vi "Execute.Initialize.vi"(8 "error in (no error)":errorcluster, 11 "Cluster":T1={"Events.State"=refnum, "Events.Test Result"=refnum, "Events.Progress"=refnum, "INI.Settings"={"Build Location"=path "C:/Simple Sequence Editor/SequenceRepo", "LoggingLocation"=path "", "Sequence.AbortChannel"="", "Sequence.IterationInfoChannel"="", "Sequence.DurationChannel"="", "Sequence.StepInfoChannel"="", "Sequence.SkipChannel"="", "PlotChannels"=[], "Sequence.InitializeScript"=path "C:/Simple Sequence Editor/SequenceRepo", "Sequence.CleanupScript"=path "", "Log.DefaultRate"=0.0}, "NIVS.AlarmManager"=refnum, "NIVS.BaseLogPath"=path "", "NIVS.DataLogManagerRef"=refnum, "NIVS.DataLogSpecRef"=refnum, "NIVS.Deployed"=FALSE, "NIVS.Events"={"SequenceEvent"=refnum, "SystemChangeEvent"=refnum, "WorkspaceEvent"=refnum}, "NIVS.GatewayIPAddress"="", "NIVS.DataLogGUID"="", "NIVS.ProfileCallback"=refnum, "NIVS.ProfileRef"=refnum, "NIVS.SequenceState"=enum."Idle", "NIVS.SystemDefinitionFile"=path "", "NIVS.SystemStateRefs"={"CustDatRef"=refnum, "EvtRef"=refnum, "Target State User Event"=refnum}, "NIVS.WorkspaceManager"=refnum, "NIVS.EventLogGUID"="", "NIVS.EventLogManagerRef"=refnum, "NIVS.EventLogSpecRef"=refnum, "NIVS.BaseToolPath"=path "", "Restart.Path"=path "", "Sequence.#ofColumns"=0, "Sequence.Iterations"=0, "Sequence.Channels"=[], "Sequence.ValidConfig?"=FALSE, "Station.ID"="", "UDP.Queue"=refnum, "UI.Abort"=refnum, "UI.Alarms"=refnum, "UI.Apply"=refnum, "UI.Back"=refnum, "UI.BaseFileName"=refnum, "UI.CurrentIteration"=refnum, "UI.CurrentStep"=refnum, "UI.CyclicFrequency"=refnum, "UI.Description"=refnum, "UI.DelayTime"=refnum, "UI.DisableAlarms"=refnum, "UI.Duration"=refnum, "UI.EnableLogging"=refnum, "UI.EnableState"=refnum, "UI.High"=refnum, "UI.LogChannels"=refnum, "UI.Low"=refnum, "UI.MonitoredVariable"=refnum, "UI.Next"=refnum, "UI.NumberOfCycles"=refnum, "UI.OperatorName"=refnum, "UI.Pause"=refnum, "UI.Profile"=refnum, "UI.Revert"=refnum, "UI.Skip"=refnum, "UI.Start"=refnum, "UI.StartIteration"=refnum, "UI.StartStep"=refnum, "UI.TabControl"=refnum, "UI.TotalIterations"=refnum, "UI.WaveformDefinition"=refnum, "UI.WaveformPreview"=refnum, "UI.WorkOrderNumber"=refnum, "UI.Chart"=refnum, "UI.Status"=refnum, "UI.DataView"=refnum, "UI.Table"=refnum, "UI.Multihead"=refnum, "UI.ToolTab"=refnum, "UI.Result"=refnum, "UI.Log Path"=refnum, "UI.ReportPath"=refnum, "UI.RestartPath"=refnum, "UI.AlarmLog"=refnum}) -> (0 "error out":errorcluster)   [LabVIEW 2015, in "Single Station Execution.lvlib"]
uses:
  Single Station Execution.lvlib
  Types/Main.StateVariables.ctl
  Types/INI.Settings.ctl
  <vilib>/NI Veristand/Execution/AlarmManager/AlarmManagerAPI.ctl
  NationalInstruments.VeriStand.ClientAPI
  <vilib>/NI Veristand/Execution/DataLogging/IDataLogging Ref.ctl
  <vilib>/NI Veristand/Execution/DataLogging/DataLoggingSpecification Ref.ctl
  Types/Execute.UserEventRefs.ctl
  <vilib>/NI Veristand/Execution/Workspace/SystemStateRegEventRef.ctl
  <vilib>/NI Veristand/Execution/Workspace/Target State Info.ctl
  <vilib>/NI Veristand/Execution/Workspace/Target State.ctl
  Types/Execution.SequenceState.ctl
  <vilib>/NI Veristand/Execution/Workspace/SystemStateEventRef.ctl
  <vilib>/NI Veristand/Execution/Workspace/WorkspaceAPI.ctl
  Types/UDPEngine.QueueCluster.ctl
  Types/UDPEngine.State.ctl
  <vilib>/NI Veristand/Execution/Workspace/NI_VS Workspace ExecutionAPI.lvlib
  <vilib>/NI Veristand/Execution/DataLogging/NI_VS Data Logging API.lvlib
  NationalInstruments.VeriStand.RealTimeSequenceDefinitionApi
  <vilib>/NI Veristand/Execution/AlarmManager/NI_VS AlarmManager ExecutionAPI.lvlib
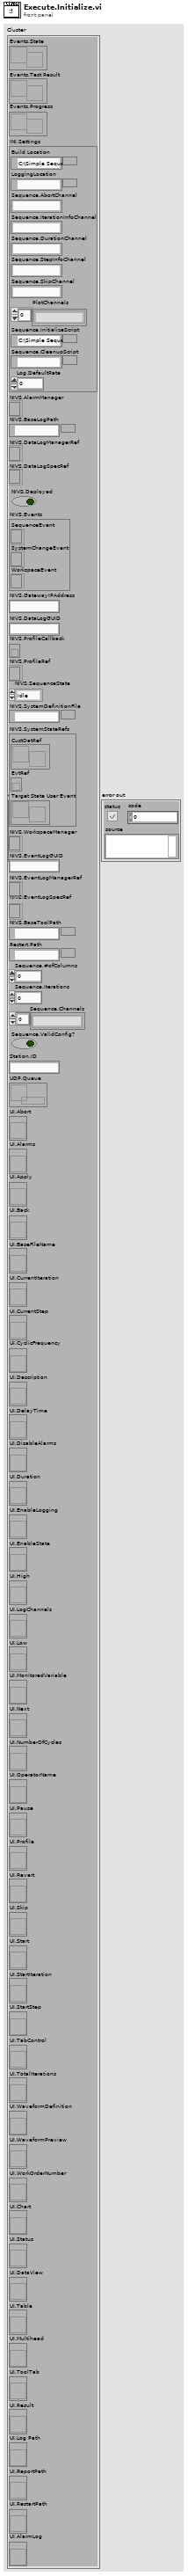
[diagram p1: front panel]
types:
  T1 = typedef "Single Station Execution.lvlib/Main.StateVariables.ctl" = cluster{"Events.State":refnum<user-event>, "Events.Test Result":refnum<user-event>, "Events.Progress":refnum<user-event>, "INI.Settings":T2, "NIVS.AlarmManager":T3, "NIVS.BaseLogPath":path, "NIVS.DataLogManagerRef":T4, "NIVS.DataLogSpecRef":T5, "NIVS.Deployed":bool, "NIVS.Events":T6, "NIVS.GatewayIPAddress":string, "NIVS.DataLogGUID":string, "NIVS.ProfileCallback":refnum<k27>, "NIVS.ProfileRef":refnum<k24>, "NIVS.SequenceState":T8, "NIVS.SystemDefinitionFile":path, "NIVS.SystemStateRefs":T9, "NIVS.WorkspaceManager":T10, "NIVS.EventLogGUID":string, "NIVS.EventLogManagerRef":T4, "NIVS.EventLogSpecRef":T5, "NIVS.BaseToolPath":path, "Restart.Path":path, "Sequence.#ofColumns":i32, "Sequence.Iterations":u32, "Sequence.Channels":string[], "Sequence.ValidConfig?":bool, "Station.ID":string, "UDP.Queue":refnum<queue>, "UI.Abort":refnum<vi>, "UI.Alarms":refnum<vi>, "UI.Apply":refnum<vi>, "UI.Back":refnum<vi>, "UI.BaseFileName":refnum<vi>, "UI.CurrentIteration":refnum<vi>, "UI.CurrentStep":refnum<vi>, "UI.CyclicFrequency":refnum<vi>, "UI.Description":refnum<vi>, "UI.DelayTime":refnum<vi>, "UI.DisableAlarms":refnum<vi>, "UI.Duration":refnum<vi>, "UI.EnableLogging":refnum<vi>, "UI.EnableState":refnum<vi>, "UI.High":refnum<vi>, "UI.LogChannels":refnum<vi>, "UI.Low":refnum<vi>, "UI.MonitoredVariable":refnum<vi>, "UI.Next":refnum<vi>, "UI.NumberOfCycles":refnum<vi>, "UI.OperatorName":refnum<vi>, "UI.Pause":refnum<vi>, "UI.Profile":refnum<vi>, "UI.Revert":refnum<vi>, "UI.Skip":refnum<vi>, "UI.Start":refnum<vi>, "UI.StartIteration":refnum<vi>, "UI.StartStep":refnum<vi>, "UI.TabControl":refnum<vi>, "UI.TotalIterations":refnum<vi>, "UI.WaveformDefinition":refnum<vi>, "UI.WaveformPreview":refnum<vi>, "UI.WorkOrderNumber":refnum<vi>, "UI.Chart":refnum<vi>, "UI.Status":refnum<vi>, "UI.DataView":refnum<vi>, "UI.Table":refnum<vi>, "UI.Multihead":refnum<vi>, "UI.ToolTab":refnum<vi>, "UI.Result":refnum<vi>, "UI.Log Path":refnum<vi>, "UI.ReportPath":refnum<vi>, "UI.RestartPath":refnum<vi>, "UI.AlarmLog":refnum<vi>}
  T2 = typedef "Single Station Execution.lvlib/INI.Settings.ctl" = cluster{"Build Location":path, "LoggingLocation":path, "Sequence.AbortChannel":string, "Sequence.IterationInfoChannel":string, "Sequence.DurationChannel":string, "Sequence.StepInfoChannel":string, "Sequence.SkipChannel":string, "PlotChannels":string[], "Sequence.InitializeScript":path, "Sequence.CleanupScript":path, "Log.DefaultRate":dbl}
  T3 = typedef "NI_VS AlarmManager ExecutionAPI.lvlib/AlarmManagerAPI.ctl" = refnum<k24>
  T4 = typedef "NI_VS Data Logging API.lvlib/IDataLogging Ref.ctl" = refnum<k24>
  T5 = typedef "NI_VS Data Logging API.lvlib/DataLoggingSpecification Ref.ctl" = refnum<k24>
  T6 = typedef "Single Station Execution.lvlib/Execute.UserEventRefs.ctl" = cluster{"SequenceEvent":refnum<event-registration>, "SystemChangeEvent":T7, "WorkspaceEvent":refnum<event-registration>}
  T7 = typedef "NI_VS Workspace ExecutionAPI.lvlib/SystemStateRegEventRef.ctl" = refnum<event-registration>
  T8 = typedef "Single Station Execution.lvlib/Execution.SequenceState.ctl" = enum16{"Idle", "Initializing", "Running", "Paused", "Finalizing", "Complete"}
  T9 = typedef "NI_VS Workspace ExecutionAPI.lvlib/SystemStateEventRef.ctl" = cluster{"CustDatRef":refnum<user-event>, "EvtRef":refnum<k27>, "Target State User Event":refnum<user-event>}
  T10 = typedef "NI_VS Workspace ExecutionAPI.lvlib/WorkspaceAPI.ctl" = refnum<k24>
  T11 = enum8{"Enabled", "Disabled", "Disabled and Grayed Out"}
  T12 = enum16{"Channels (No System Channel)", "Aliases", "All"}
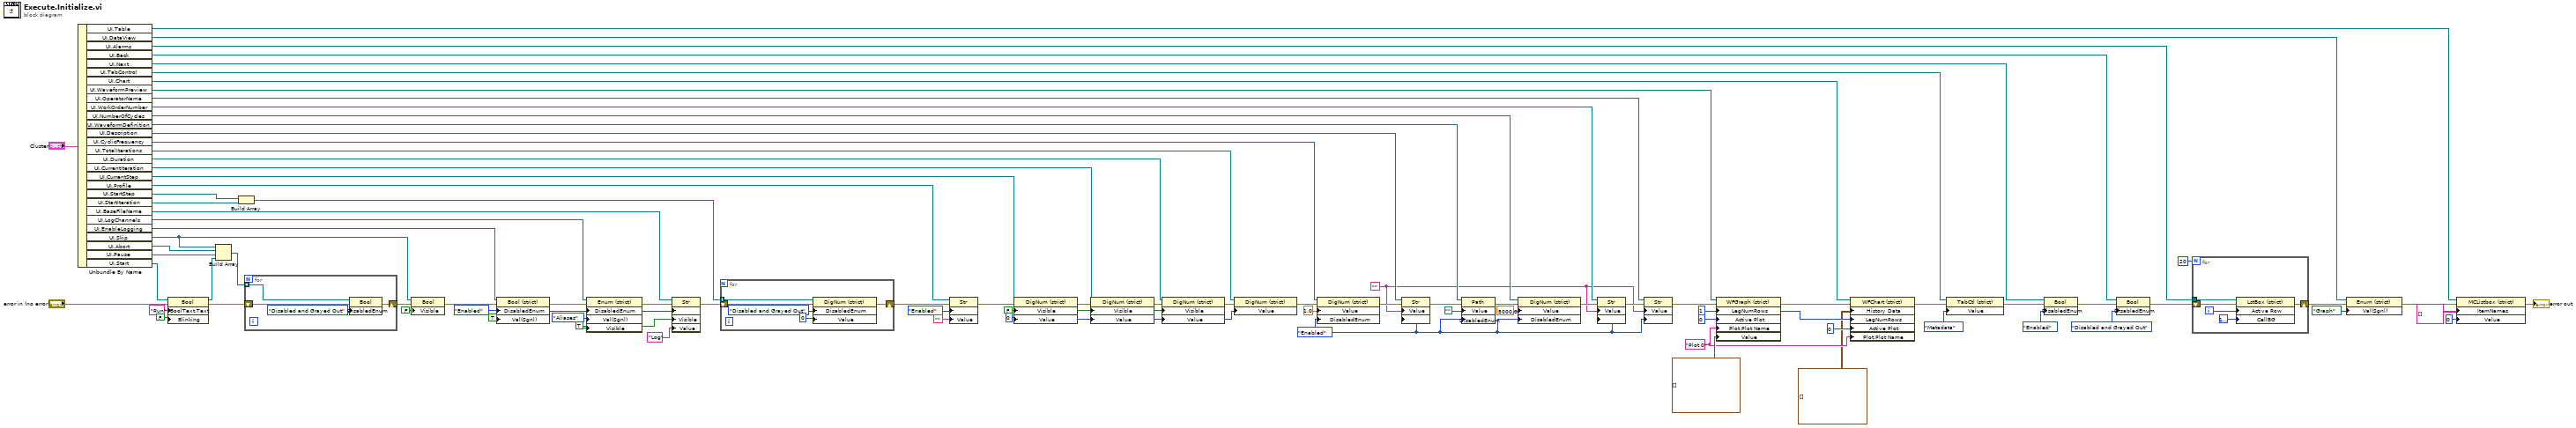
[diagram p0: block diagram]
diagram:
  w20 = T11."Enabled" ("Disabled")
  w14 = "Plot 0" ("Plot.Plot Name")
  w16 = u32 1 ("Legend:Number of Rows")
  w34 = ""
  w50 = u32 0 ("Value")
  w51 = FALSE ("Visible")
  w1 = TRUE ("Visible")
  w74 = T11."Enabled" ("Disabled")
  n1 = Unbundle By Name("Cluster") -> ("UI.Table"=w4:refnum<vi>, "UI.DataView"=w8:refnum<vi>, "UI.Alarms"=w12:refnum<vi>, "UI.Back"=w25:refnum<vi>, "UI.Next"=w26:refnum<vi>, "UI.TabControl"=w27:refnum<vi>, "UI.Chart"=w17:refnum<vi>, "UI.WaveformPreview"=w31:refnum<vi>, "UI.OperatorName"=w38:refnum<vi>, "UI.WorkOrderNumber"=w39:refnum<vi>, "UI.NumberOfCycles"=w40:refnum<vi>, "UI.WaveformDefinition"=w41:refnum<vi>, "UI.Description"=w42:refnum<vi>, "UI.CyclicFrequency"=w43:refnum<vi>, "UI.TotalIterations"=w67:refnum<vi>, "UI.Duration"=w52:refnum<vi>, "UI.CurrentIteration"=w69:refnum<vi>, "UI.CurrentStep"=w70:refnum<vi>, "UI.Profile"=w89:refnum<vi>, "UI.StartStep"=w86:refnum<vi>, "UI.StartIteration"=w85:refnum<vi>, "UI.BaseFileName"=w75:refnum<vi>, "UI.LogChannels"=w82:refnum<vi>, "UI.EnableLogging"=w81:refnum<vi>, "UI.Skip"=w62:refnum<vi>, "UI.Abort"=w78:refnum<vi>, "UI.Pause"=w79:refnum<vi>, "UI.Start"=w56:refnum<vi>)
  n2 = property class="Bool"(reference=w56, error in="error in (no error)", "BoolText.Text"="Run" ("Boolean Text.Text"), "Blinking"=FALSE) -> (reference out=w55:refnum<vi>, error out=w59:errorcluster)
  n3 = Build Array(w62, w78, w79, w55) -> (w80:refnum<vi>[])
  n4 = Build Array(w86, w85) -> (w87:refnum<vi>[])
  n5 = for {
    tunnel: w80 -> [w93] mode=indexing
    shift-right: [w91] -> w64
    shift-left: w59 -> [w90]
    n6 = property class="Bool"(reference=w93, error in=w90, "DisabledEnum"=T11."Disabled and Grayed Out" ("Disabled")) -> (error out=w91:errorcluster)  [unwired: 1 out]
  }
  n7 = property class="Bool"(reference=w62, error in=w64, "Visible"=FALSE) -> (error out=w63:errorcluster)  [unwired: 1 out]
  n8 = property class="Bool (strict)"(reference=w81, error in=w63, "DisabledEnum"=w74, "Val(Sgnl)"=TRUE ("Value (Signaling)")) -> (error out=w83:errorcluster)  [unwired: 1 out]
  n9 = property class="Enum (strict)"(reference=w82, error in=w83, "DisabledEnum"=w74, "Val(Sgnl)"=T12."Aliases" ("Value (Signaling)"), "Visible"=w1) -> (error out=w73:errorcluster)  [unwired: 1 out]
  n10 = property class="Str"(reference=w75, error in=w73, "DisabledEnum"=w74, "Visible"=w1, "Value"="Log") -> (error out=w72:errorcluster)  [unwired: 1 out]
  n11 = for {
    tunnel: w87 -> [w98] mode=indexing
    shift-right: [w96] -> w88
    shift-left: w72 -> [w95]
    n12 = property class="DigNum (strict)"(reference=w98, error in=w95, "DisabledEnum"=T11."Disabled and Grayed Out" ("Disabled"), "Value"=u32 0) -> (error out=w96:errorcluster)  [unwired: 1 out]
  }
  n13 = property class="Str"(reference=w89, error in=w88, "DisabledEnum"=T11."Enabled" ("Disabled"), "Value"="") -> (error out=w49:errorcluster)  [unwired: 1 out]
  n14 = property class="DigNum (strict)"(reference=w70, error in=w49, "Visible"=w51, "Value"=w50) -> (error out=w68:errorcluster)  [unwired: 1 out]
  n15 = property class="DigNum (strict)"(reference=w69, error in=w68, "Visible"=w51, "Value"=w50) -> (error out=w54:errorcluster)  [unwired: 1 out]
  n16 = property class="DigNum (strict)"(reference=w52, error in=w54, "Visible"=w51, "Value"=w50) -> (error out=w53:errorcluster)  [unwired: 1 out]
  n17 = property class="DigNum (strict)"(reference=w67, error in=w53, "Value"=w50) -> (error out=w37:errorcluster)  [unwired: 1 out]
  n18 = property class="DigNum (strict)"(reference=w43, error in=w37, "Value"=1.0, "DisabledEnum"=w20) -> (error out=w44:errorcluster)  [unwired: 1 out]
  n19 = property class="Str"(reference=w42, error in=w44, "Value"=w34, "DisabledEnum"=w20) -> (error out=w48:errorcluster)  [unwired: 1 out]
  n20 = property class="Path"(reference=w41, error in=w48, "Value"=path "", "DisabledEnum"=w20) -> (error out=w46:errorcluster)  [unwired: 1 out]
  n21 = property class="DigNum (strict)"(reference=w40, error in=w46, "Value"=5000.0, "DisabledEnum"=w20) -> (error out=w47:errorcluster)  [unwired: 1 out]
  n22 = property class="Str"(reference=w39, error in=w47, "Value"=w34, "DisabledEnum"=w20) -> (error out=w45:errorcluster)  [unwired: 1 out]
  n23 = property class="Str"(reference=w38, error in=w45, "Value"=w34, "DisabledEnum"=w20) -> (error out=w32:errorcluster)  [unwired: 1 out]
  n24 = property class="WFGraph (strict)"(reference=w31, error in=w32, "LegNumRows"=w16, "Active Plot"=u32 0, "Plot.Plot Name"=w14, "Value"=waveform(dbl)[] []) -> (error out=w19:errorcluster)  [unwired: 1 out]
  n25 = property class="WFChart (strict)"(reference=w17, error in=w19, "History Data"=waveform(dbl)[][] [], "LegNumRows"=w16, "Active Plot"=u32 0, "Plot.Plot Name"=w14) -> (error out=w18:errorcluster)  [unwired: 1 out]
  n26 = property class="TabCtl (strict)"(reference=w27, error in=w18, "Value"=enum32{"Metadata", "Alarms", "Execution"}."Metadata") -> (error out=w28:errorcluster)  [unwired: 1 out]
  n27 = property class="Bool"(reference=w26, error in=w28, "DisabledEnum"=T11."Enabled" ("Disabled")) -> (error out=w29:errorcluster)  [unwired: 1 out]
  n28 = property class="Bool"(reference=w25, error in=w29, "DisabledEnum"=T11."Disabled and Grayed Out" ("Disabled")) -> (error out=w13:errorcluster)  [unwired: 1 out]
  n29 = for {
    N: 20 -> [_]
    shift-right: [w102] -> w9
    shift-left: w13 -> [w103]
    tunnel: w12 -> [w101]
    i -> [w100]
    n30 = property class="LstBox (strict)"(reference=w101, error in=w103, "Active Row"=w100, "CellBG"=u32 16777216) -> (error out=w102:errorcluster)  [unwired: 1 out]
  }
  n31 = property class="Enum (strict)"(reference=w8, error in=w9, "Val(Sgnl)"=enum16{"Graph", "Table"}."Graph" ("Value (Signaling)")) -> (error out=w6:errorcluster)  [unwired: 1 out]
  n32 = property class="MCListbox (strict)"(reference=w4, error in=w6, "ItemNames"=string[][] [] ("Item Names"), "Value"=0) -> (error out=→"error out":errorcluster)  [unwired: 1 out]
